vi "Query numeric.vi"(8 "Error In":errorcluster, 10 "Query String":string, 11 "VISA resource name":refnum<visa-resource-name>) -> (0 "Error Out":errorcluster, 1 "data string out":string, 2 "Numeric":dbl, 3 "VISA resource name out":refnum<visa-resource-name>)   [LabVIEW 2021]
uses:
  VISA  Send Receive.vi
  Simple VISA Reader/Simple VISA Reader Driver.lvclass
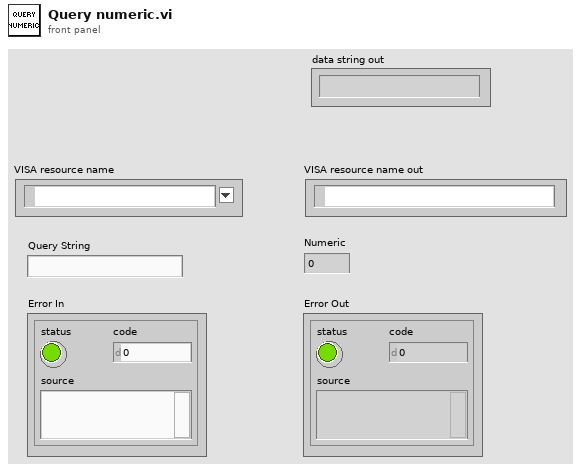
[diagram p1: front panel]
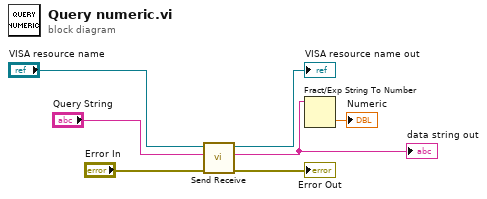
[diagram p0: block diagram]
diagram:
  n1 = call-poly "Send Receive.vi"("error in (no error)"="Error In", "data string in"="Query String", "VISA Resource Name"="VISA resource name") -> ("error out"=→"Error Out":errorcluster, "data string out"=w2:string, "VISA Resource Name Out"=→"VISA resource name out":refnum<visa-resource-name>)  [unwired: 6 in]
  "data string out" <- w2
  n2 = Fract/Exp String To Number(string=w2) -> (number=→"Numeric":dbl)  [unwired: 3 in, 1 out]
